vi "Create File.vi"(8 "error in":errorcluster, 11 "Log in":refnum<class "Log.lvclass">) -> (0 "error out":errorcluster, 3 "Log out":refnum<class "Log.lvclass">)   [LabVIEW 2017, in "Report_lib.lvlib" / "Log.lvclass"]
doc: "This Dynamic SubVI use for further replace \nsuch SubVI in child classes and create new text file\nFor inheritance in child classes"
uses:
  Log.lvclass
  Log.lvclass/Log.ctl
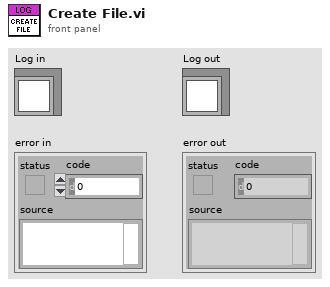
[diagram p1: front panel]
types:
  T1 = enum16{"open", "replace", "create", "open or create", "replace or create", "replace or create with confirmation"}
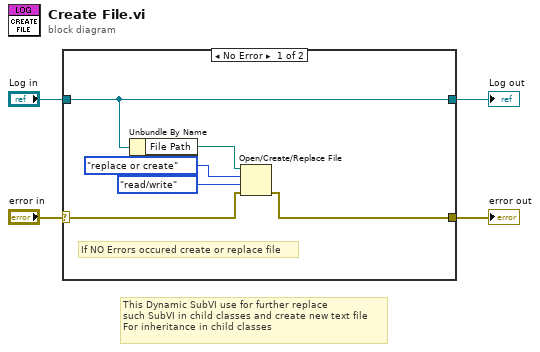
[diagram p0: block diagram]
diagram:
  # "This Dynamic SubVI use for further replace \nsuch SubVI in child classes and create new text file\nFor inheritance in child classes"
  n1 = case shown="No Error" "error in" {
    selector: "error in" -> [w8 w12]
    tunnel: [w7 w12] -> w3
    tunnel: [w5 w11] -> w1
    tunnel: "Log in" -> [w5 w11]
    frame No Error {
      # "If NO Errors occured create or replace file"
      n2 = Unbundle By Name(w5) -> ("File Path"=w6:path)
      n3 = Open/Create/Replace File(file path (use dialog)=w6, error in=w8, operation (0:open)=T1."replace or create", access (0:read/write)=enum16{"read/write", "read-only", "write-only"}."read/write") -> (error out=w7:errorcluster)  [unwired: 2 in, 2 out]
    }
    frame Error {
    }
  }
  "error out" <- w3
  "Log out" <- w1
